vi "StickyButton.vi"(1 "Time threshold (ms)":u32, 2 "Button Input":bool) -> (0 "Sticky Button":bool)   [LabVIEW 2020]
doc: "The input stays true for a certain number of seconds after release and it starts as false. \n\nButton input (bool):\nInput signal\n\nTime threshold (ms):\nAmount of time ButtonInput stays true after release \n\nSticky Button (bool):\nOutput"
uses:
  d4953c67-f53d-41fa-97a7-851cc2dfed5b.vi
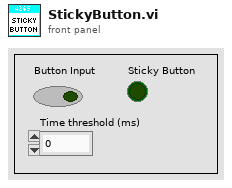
[diagram p1: front panel]
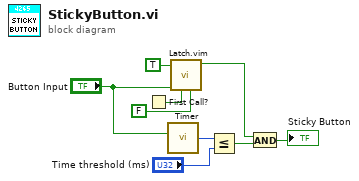
[diagram p0: block diagram]
diagram:
  n1 = First Call?() -> (First Call?: T/F=w6:bool)
  n2 = call "Timer.vi"("Reset Timer"="Button Input") -> ("Time (ms)"=w9:u32)
  n3 = call "Latch.vim"("Default Value"=FALSE, "Reset"=w6, "Latch Signal"="Button Input", "Latch Value"=TRUE) -> ("Latched"=w4:bool)  [unwired: 7 in]
  n4 = Less Or Equal?(x=w9, y="Time threshold (ms)") -> (x <= y?=w5:bool)
  n5 = And(x=w4, y=w5) -> (x .and. y?=→"Sticky Button":bool)
